vi "sm string write and increment.vi"(9 "Identifier":string, 10 "String in":string, 11 "Shared memory cluster input":T1) -> (3 "Shared memory cluster output":T1)   [LabVIEW 2019, in "linuxSharedMemory.lvlib"]
uses:
  linuxSharedMemory.lvlib
  controls/sm_cluster.ctl
  <vilib>/NI/NI Linux RT IPC/Shared Memory/Pointer Operations/Write String.vi
  <vilib>/NI/NI Linux RT IPC/Shared Memory/Pointer Operations/In Place Write String.vi
  <vilib>/NI/NI Linux RT IPC/Shared Memory/Linux RT IPC.Shared Memory.lvlib
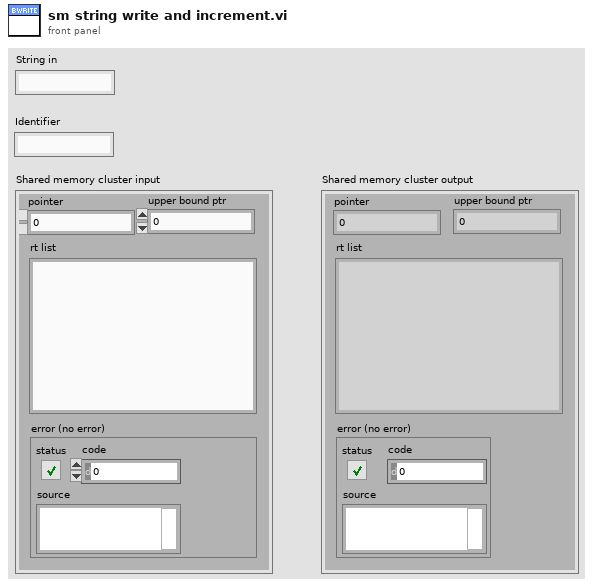
[diagram p1: front panel]
types:
  T1 = typedef "linuxSharedMemory.lvlib/sm_cluster.ctl" = cluster{"rt list":string, "error (no error)":errorcluster, "pointer":u64, "upper bound ptr":u64}
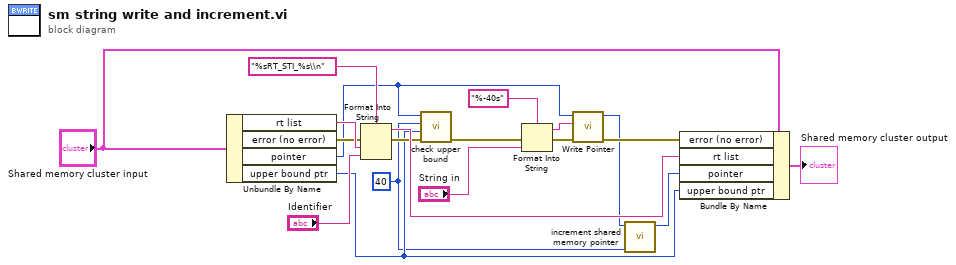
[diagram p0: block diagram]
diagram:
  w6 = 40
  n1 = Unbundle By Name("Shared memory cluster input") -> ("rt list"=w15:string, "error (no error)"=w13:errorcluster, "pointer"=w8:u64, "upper bound ptr"=w10:u64)
  n2 = Format Into String(format string="%sRT_STI_%s\\n", error in=w13, w15, "Identifier") -> (resulting string=w14:string, error out=w12:errorcluster)  [unwired: 1 in]
  n3 = call "check upper bound.vi"("error in (no error)"=w12, "ptr upper bound (inclusive)"=w10, "size"=w6, "ptr in"=w8) -> ("error out"=w3:errorcluster)  [unwired: 7 in]
  n4 = Format Into String(format string="%-40s", error in=w3, "String in") -> (resulting string=w1:string, error out=w2:errorcluster)  [unwired: 1 in]
  n5 = call-poly <vilib>:"Write Pointer.vi"("error in (no error)"=w2, "string in"=w1, "pointer in"=w8) -> ("error out"=w9:errorcluster, "pointer out"=w7:u64)  [unwired: 5 in, 2 out]
  n6 = call "increment shared memory pointer.vi"("Increment value"=w6, "Shared Memory PTR in"=w7) -> ("Shared Memory PTR out"=w11:u64)  [unwired: 9 in]
  n7 = Bundle By Name(cluster="Shared memory cluster input", "error (no error)"=w9, "rt list"=w14, "pointer"=w11, "upper bound ptr"=w10) -> (→"Shared memory cluster output":T1)
